vi "3.3.vi"() -> ()   [LabVIEW 2017]
panel:
  in  "偏移量3":dbl
  out "数值":dbl
  out "子字符串 2":string
  out "子字符串 1":string
  in  "长度2":dbl
  in  "偏移量2":dbl
  in  "长度1":dbl
  in  "偏移量1":dbl
  in  "输入字符串":string
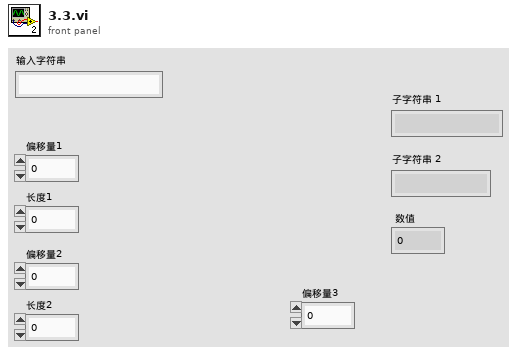
[diagram p1: front panel]
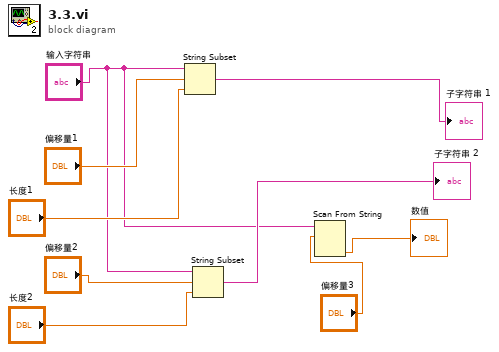
[diagram p0: block diagram]
diagram:
  n1 = String Subset(string="输入字符串", offset (0)="偏移量1", length (rest)="长度1") -> (substring=→"子字符串 1":string)
  n2 = String Subset(string="输入字符串", offset (0)="偏移量2", length (rest)="长度2") -> (substring=→"子字符串 2":string)
  n3 = Scan From String(input string="输入字符串", initial scan location="偏移量3") -> (output 1=→"数值":dbl)  [unwired: 3 in, 3 out]
